vi "Configure Trigger (SPI).vi"(0 "VISA resource name":refnum<visa-resource-name>, 1 "Trigger On (1:MOSI)":u16(ring)=1 items=["MISO", "MOSI"], 2 "MOSI":T2={"MOSI Source (2:Channel3)"=2, "MOSI Polarity (0:Active High)"=0, "MOSI Data Threshold(0)"=0.0} {"MOSI Polarity (0:Active High)" items=["Active High", "Active Low"]; "MOSI Source (2:Channel3)" items=["Channel1", "Channel2", "Channel3", "Channel4"]}, 3 "MISO":T1={"MISO Source (3:Channel4)"=3, "MISO Polarity (0:Active High)"=0, "MISO Data Threshold(0)"=0.0} {"MISO Polarity (0:Active High)" items=["Active High", "Active Low"]; "MISO Source (3:Channel4)" items=["Channel1", "Channel2", "Channel3", "Channel4"]}, 5 "SS Configure":T4 {"SS Polarity (0:Active High)" items=["Active High", "Active Low"]; "SS Source (0:Channel1)" items=["Channel1", "Channel2", "Channel3", "Channel4"]}, 7 "SCLK Configure":T3={"SCLK Source (1:Channel2)"=1, "SCLK Threshold (0.0V)"=0.0, "SCLK Polarity (0:Falling)"=0} {"SCLK Polarity (0:Falling)" items=["Falling", "Rising"]; "SCLK Source (1:Channel2)" items=["Channel1", "Channel2", "Channel3", "Channel4"]}, 9 "Start Position(0)":u16, 11 "error in (no error)":errorcluster, 12 "Identifier Value":string) -> (4 "VISA resource name out":refnum<visa-resource-name>, 15 "error out":errorcluster)   [LabVIEW 2015, in "Tektronix 7000 Series.lvlib"]
doc: "Configures SPI trigger settings for an oscilloscope.A SPI trigger occurs when a Serial Peripheral Interface signal is found.\n\n<b>Note:</b>\nOnly DPO7000 series oscilloscopes supports this Trigger."
uses:
  <instrlib>/Tektronix 7000 Series/Tektronix 7000 Series.lvlib
panel:
  # "msb"
  # "lsb"
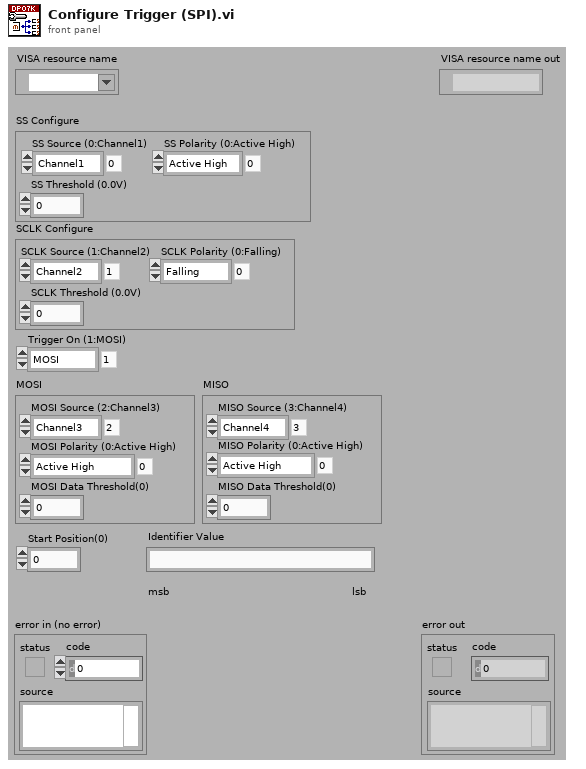
[diagram p1: front panel]
types:
  T1 = cluster{"MISO Source (3:Channel4)":u16, "MISO Polarity (0:Active High)":u16, "MISO Data Threshold(0)":dbl}
  T2 = cluster{"MOSI Source (2:Channel3)":u16, "MOSI Polarity (0:Active High)":u16, "MOSI Data Threshold(0)":dbl}
  T3 = cluster{"SCLK Source (1:Channel2)":u16, "SCLK Threshold (0.0V)":dbl, "SCLK Polarity (0:Falling)":u16}
  T4 = cluster{"SS Source (0:Channel1)":u16, "SS Threshold (0.0V)":dbl, "SS Polarity (0:Active High)":u16}
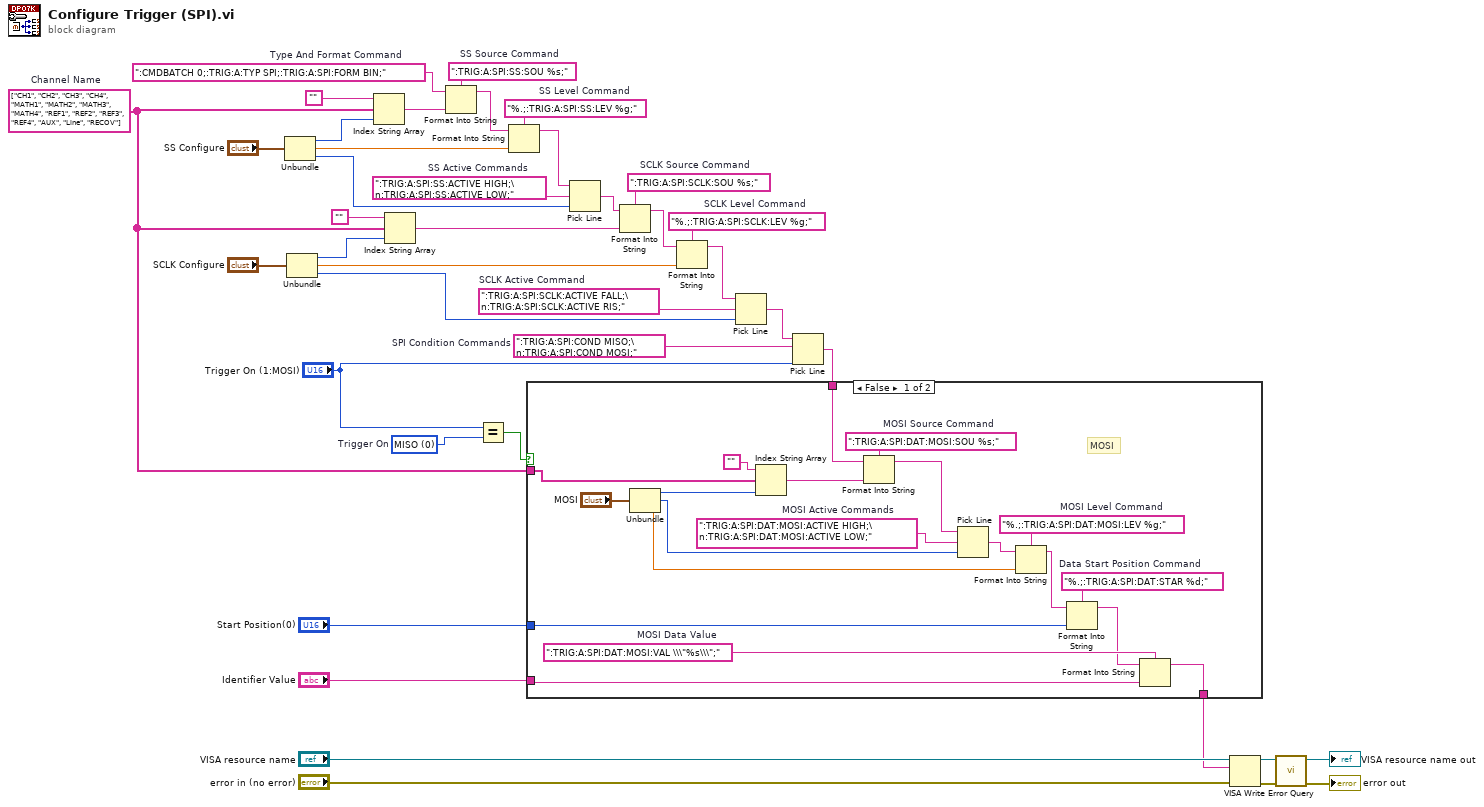
[diagram p0: block diagram]
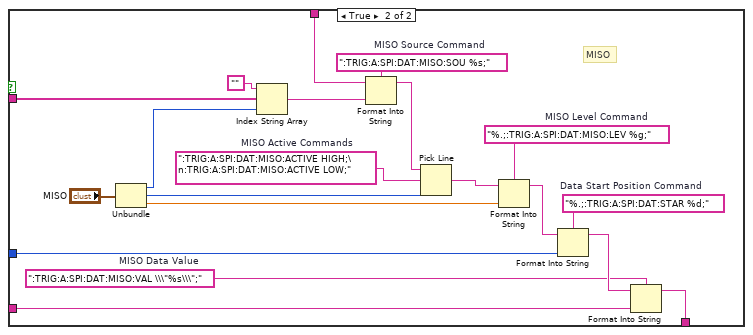
[diagram p2: hidden frame]
diagram:
  w14 = u16 0 items=["MISO", "MOSI"]  # Trigger On
  w15 = ":TRIG:A:SPI:COND MISO;\n:TRIG:A:SPI:COND MOSI;"  # SPI Condition Commands
  w17 = ":TRIG:A:SPI:SCLK:ACTIVE FALL;\n:TRIG:A:SPI:SCLK:ACTIVE RIS;"  # SCLK Active Command
  w21 = "%.;:TRIG:A:SPI:SCLK:LEV %g;"  # SCLK Level Command
  w23 = ":TRIG:A:SPI:SCLK:SOU %s;"  # SCLK Source Command
  w30 = ":TRIG:A:SPI:SS:ACTIVE HIGH;\n:TRIG:A:SPI:SS:ACTIVE LOW;"  # SS Active Commands
  w32 = "%.;:TRIG:A:SPI:SS:LEV %g;"  # SS Level Command
  w35 = ":TRIG:A:SPI:SS:SOU %s;"  # SS Source Command
  w11 = string[] ["CH1", "CH2", "CH3", "CH4", "MATH1", "MATH2", "MATH3", "MATH4", "REF1", "REF2", "REF3", "REF4", "AUX", "Line", "RECOV"]  # Channel Name
  w36 = ":CMDBATCH 0;:TRIG:A:TYP SPI;:TRIG:A:SPI:FORM BIN;"  # Type And Format Command
  n1 = Unbundle("SS Configure") -> ("SS Source (0:Channel1)"=w38:u16, "SS Threshold (0.0V)"=w34:dbl, "SS Polarity (0:Active High)"=w29:u16)
  n2 = Unbundle("SCLK Configure") -> ("SCLK Source (1:Channel2)"=w26:u16, "SCLK Threshold (0.0V)"=w22:dbl, "SCLK Polarity (0:Falling)"=w18:u16)
  n3 = Index String Array(1:w38, 2:w11, 3:"") -> (0:w37:string)
  n4 = Index String Array(1:w26, 2:w11, 3:"") -> (0:w25:string)
  n5 = Format Into String(format string=w35, initial string=w36, w37) -> (resulting string=w33:string)  [unwired: 1 in, 1 out]
  n6 = Equal?(x="Trigger On (1:MOSI)", y=w14) -> (x = y?=w12:bool)
  n7 = Format Into String(format string=w32, initial string=w33, w34) -> (resulting string=w31:string)  [unwired: 1 in, 1 out]
  n8 = Pick Line(string ("")=w31, multi-line string=w30, line index=w29) -> (output string=w24:string)
  n9 = Format Into String(format string=w23, initial string=w24, w25) -> (resulting string=w20:string)  [unwired: 1 in, 1 out]
  n10 = Format Into String(format string=w21, initial string=w20, w22) -> (resulting string=w19:string)  [unwired: 1 in, 1 out]
  n11 = Pick Line(string ("")=w19, multi-line string=w17, line index=w18) -> (output string=w16:string)
  n12 = Pick Line(string ("")=w16, multi-line string=w15, line index="Trigger On (1:MOSI)") -> (output string=w10:string)
  n13 = case shown="False" w12 {
    tunnel: w11 -> [w45 w77]
    tunnel: w10 -> [w44 w75]
    tunnel: "Start Position(0)" -> [w43 w68]
    tunnel: "Identifier Value" -> [w42 w63]
    tunnel: [w41 w62] -> w1
    frame False {
      w60 = ":TRIG:A:SPI:DAT:MOSI:VAL \\\"%s\\\";"  # MOSI Data Value
      w58 = "%.;:TRIG:A:SPI:DAT:STAR %d;"  # Data Start Position Command
      w56 = "%.;:TRIG:A:SPI:DAT:MOSI:LEV %g;"  # MOSI Level Command
      w51 = ":TRIG:A:SPI:DAT:MOSI:ACTIVE HIGH;\n:TRIG:A:SPI:DAT:MOSI:ACTIVE LOW;"  # MOSI Active Commands
      w50 = ":TRIG:A:SPI:DAT:MOSI:SOU %s;"  # MOSI Source Command
      # "MOSI"
      n14 = Unbundle("MOSI") -> ("MOSI Source (2:Channel3)"=w48:u16, "MOSI Polarity (0:Active High)"=w52:u16, "MOSI Data Threshold(0)"=w55:dbl)
      n15 = Index String Array(1:w48, 2:w45, 3:"") -> (0:w49:string)
      n16 = Format Into String(format string=w50, initial string=w44, w49) -> (resulting string=w53:string)  [unwired: 1 in, 1 out]
      n17 = Pick Line(string ("")=w53, multi-line string=w51, line index=w52) -> (output string=w54:string)
      n18 = Format Into String(format string=w56, initial string=w54, w55) -> (resulting string=w57:string)  [unwired: 1 in, 1 out]
      n19 = Format Into String(format string=w58, initial string=w57, w43) -> (resulting string=w59:string)  [unwired: 1 in, 1 out]
      n20 = Format Into String(format string=w60, initial string=w59, w42) -> (resulting string=w41:string)  [unwired: 1 in, 1 out]
    }
    frame True {
      w64 = ":TRIG:A:SPI:DAT:MISO:VAL \\\"%s\\\";"  # MISO Data Value
      w66 = "%.;:TRIG:A:SPI:DAT:STAR %d;"  # Data Start Position Command
      w69 = "%.;:TRIG:A:SPI:DAT:MISO:LEV %g;"  # MISO Level Command
      w73 = ":TRIG:A:SPI:DAT:MISO:ACTIVE HIGH;\n:TRIG:A:SPI:DAT:MISO:ACTIVE LOW;"  # MISO Active Commands
      w74 = ":TRIG:A:SPI:DAT:MISO:SOU %s;"  # MISO Source Command
      # "MISO"
      n21 = Unbundle("MISO") -> ("MISO Source (3:Channel4)"=w78:u16, "MISO Polarity (0:Active High)"=w72:u16, "MISO Data Threshold(0)"=w61:dbl)
      n22 = Index String Array(1:w78, 2:w77, 3:"") -> (0:w76:string)
      n23 = Format Into String(format string=w74, initial string=w75, w76) -> (resulting string=w71:string)  [unwired: 1 in, 1 out]
      n24 = Pick Line(string ("")=w71, multi-line string=w73, line index=w72) -> (output string=w70:string)
      n25 = Format Into String(format string=w69, initial string=w70, w61) -> (resulting string=w67:string)  [unwired: 1 in, 1 out]
      n26 = Format Into String(format string=w66, initial string=w67, w68) -> (resulting string=w65:string)  [unwired: 1 in, 1 out]
      n27 = Format Into String(format string=w64, initial string=w65, w63) -> (resulting string=w62:string)  [unwired: 1 in, 1 out]
    }
  }
  n28 = VISA Write(VISA resource name="VISA resource name", write buffer=w1, error in (no error)="error in (no error)") -> (VISA resource name out=w7:refnum<visa-resource-name>, error out=w6:errorcluster)  [unwired: 1 out]
  n29 = call <instrlib>:"Error Query.vi"("error in (no error)"=w6, "VISA resource name"=w7) -> ("error out"=→"error out":errorcluster, "VISA resource name out"=→"VISA resource name out":refnum<visa-resource-name>)  [unwired: 6 in, 2 out]
